vi "2100_Test_Guardian Switch_w Config.vi"(0 "Semiconductor Module Context":T7, 1 "SMU Current Settings":T6={"OFF_Current  Range"=1e-05, "OFF_Current  Level"=-1e-05, "ON_Current  Range"=0.001, "ON_Current  Level"=0.001} {"ON_Current  Level" format="%#_6p"; "ON_Current  Range" format="%#_6p"; "OFF_Current  Level" format="%#_6p"; "OFF_Current  Range" format="%#_6p"}, 2 "Master_Register_Data_Array_In":T1 {"Address" format="%.0x"}, 3 "Set_Meas_Sense":i32(ring)=1008 items=["Local"=1008, "Remote"=1009], 5 "Script_Info":T4={"Script Name"="WalkingState", "All_Scripts"=[]}, 7 "Publishable IDs":string[](array[string])=["LowPower", "Active"], 9 "USID":T3 max=15, 11 "Error In":errorcluster, 12 "Instrument_Pins":T5={"SMU_Pins"=["RF1", "RF2", "RF3", "RF4"], "HSDIO_Pins"=["CLK", "SDA"]}, 13 "Reg_Map_Bit_Name":string="RFC_SH", 14 "Reg_Map":string[][](array[string])=[["Reg Addr(0x00)", "7", "6", "5", "4", "3", "2", "1", "0"], ["0", "SPARE", "RF3_SH", "RF2_SH", "RF1_SH", "SPARE", "RF3_RFC", "RF2_RFC", "RF1_RFC"], ["1", "SPARE[7:0]", "", "", "", "", "", "", ""], ["2", "VVAR_EN", "LCM_EN", "RFC_SH", "SPARE", "VARACTOR[3:0]", "", "", ""], ["3", "SW_CTRL1_VIRTUAL[7:0]", "", "", "", "", "", "", ""], ["4", "SW_CTRL1_SWAP", "SW_CTRL1_RBSHIFT[2:0]", "", "", "SW_CTRL1_VSID[3:0]", "", "", ""], ["5", "REG_00_VIRTUAL_MASK[7:0]", "", "", "", "", "", "", ""], ["6", "LOCK_STATUS[1:0]", "", "CLK_DITHER", "FUSES_BURNED", "CLK_IDAC_CAL[3:0]", "", "", ""], ["7", "SPARE[2:0]", "", "", "ODFT_TRIM[4:0]", "", "", "", ""], ["8", "SPARE[2:0]", "", "", "HV_TRIM[4:0]", "", "", "", ""], ["9", "TEST_MUX[2:0]", "", "", "SPARE[1:0]", "", "MEMS_BG_TC[1:0]", "", "MEMSCP_RCM"], ["A", "CP_BOOST_OVRD_EN", "SPARE[2:0]", "", "", "PS_OFF_TIMER[1:0]", "", "PS_ON_TIMER[1:0]", ""], ["0", "", "", "", "", "", "", "", ""], ["D", "Reserved[1:0]", "", "WD_HI_EVENT_CNT[5:0]", "", "", "", "", ""], ["E", "VERSION_ID[7:0]", "", "", "", "", "", "", ""], ["F", "Reserved", "COUNT_200_LSB[6:0]", "", "", "", "", "", ""], ["10", "CLK_DIV2_EN", "Spare", "ODFT_EN", "HV_HYST[4:0]", "", "", "", ""], ["0", "", "", "", "", "", "", "", ""], ["12", "SHORT_FUSE", "FUSE_BURN", "STROBE_EN", "VIO_OK", "RTH[1:0]", "", "FUSE_LOAD_MAN_EN", "FUSE_LOAD"], ["13", "RR_ACK_EN", "Reserved", "ACK_POSITION[1:0]", "", "SuBUS_DRIVE_STRENGTH[3:0]", "", "", ""], ["14", "TM_IO_EN", "TM_IO_SEL", "SuBUS_OVS[1:0]", "", "Reserved[3:0]", "", "", ""], ["15", "Reserved[4:0]", "", "", "", "", "SuBUS_VERSION_PRESENT", "SuBUS_VOLTAGE", "SuBUS_FLAVOR_DEF"], ["16", "PROG_STROBE1_DUR[7:0]", "", "", "", "", "", "", ""], ["17", "PROG_STROBE0_DUR[7:0]", "", "", "", "", "", "", ""], ["18", "Reserved[2:0]", "", "", "EFUSE_SINGLE_ADDR_SEL[4:0]", "", "", "", ""], ["19", "POLL_ADR[4:0]", "", "", "", "", "POLL_BC[2:0]", "", ""], ["1A", "SOFTWARE_RESET", "Reserved[6:0]", "", "", "", "", "", ""], ["1B", "Reserved[7:0]", "", "", "", "", "", "", ""], ["1C", "PWR_MODE_1", "PWR_MODE_0", "TRIGGER_MASK[2:0]", "", "", "TRIGGER[2:0]", "", ""], ["1D", "PRODUCT_ID[7:0]", "", "", "", "", "", "", ""], ["1E", "MANUFACTURER_ID_LSB[7:0]", "", "", "", "", "", "", ""], ["1F", "MANUFACTURER_ID_MSB[3:0]", "", "", "", "USID[3:0]", "", "", ""]]) -> (6 "Master_Register_Data_Array_Out":T1 {"Address" format="%.0x"}, 15 "Error Out":errorcluster)   [LabVIEW 2013]
uses:
  Controls/USID.ctl
  <vilib>/NI_TestStand_SemiconductorModule/NI_TestStand_Semiconductor_Module.lvlibp/PinMap/General/SemiconductorModuleContext.ctl
  Controls/Master_Reg_Data_Array.ctl
  Controls/Reg_Address_Data.ctl
  <vilib>/NI_TestStand_SemiconductorModule/NI_TestStand_Semiconductor_Module.lvlibp/PinMap/DC Power/PinsToNIDCPowerSessions.vi
  <vilib>/NI_TestStand_SemiconductorModule/NI_TestStand_Semiconductor_Module.lvlibp/PinMap/General/Publish/PublishDataDoubleFunctionalTest.vi
  <vilib>/NI_TestStand_SemiconductorModule/NI_TestStand_Semiconductor_Module.lvlibp
panel:
  out "R Array":dbl[][](array[numeric]) format="%#_6p"
  in  "Tab Control":enum32{"Test Info", "Instrument Settings"}(tab)
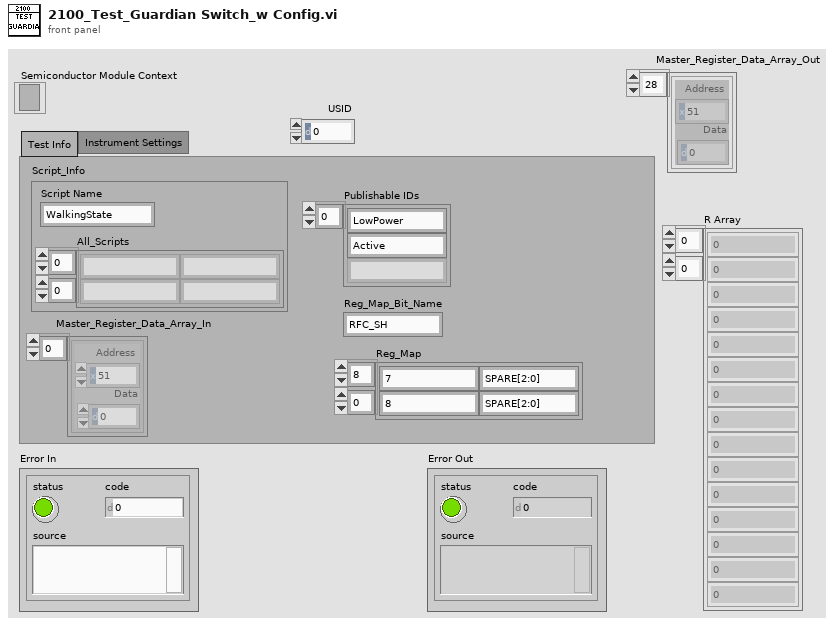
[diagram p1: front panel]
types:
  T1 = typedef "Master_Reg_Data_Array.ctl" = T2[]
  T2 = typedef "Reg_Address_Data.ctl" = cluster{"Address":u8, "Data":u8}
  T3 = typedef "USID.ctl" = u8
  T4 = cluster{"Script Name":string, "All_Scripts":string[][]}
  T5 = cluster{"SMU_Pins":string[], "HSDIO_Pins":string[]}
  T6 = cluster{"OFF_Current  Range":dbl, "OFF_Current  Level":dbl, "ON_Current  Range":dbl, "ON_Current  Level":dbl}
  T7 = typedef "NI_TestStand_Semiconductor_Module.lvlibp/SemiconductorModuleContext.ctl" = refnum<k7>
  T8 = typedef "Script Functions_Array.ctl" = enum16{"Reg_Write", "Bit_Write", "Delay", "Read", "Measure"}[]
  T9 = enum16{"Reg_Write", "Bit_Write", "Delay", "Read", "Measure"}
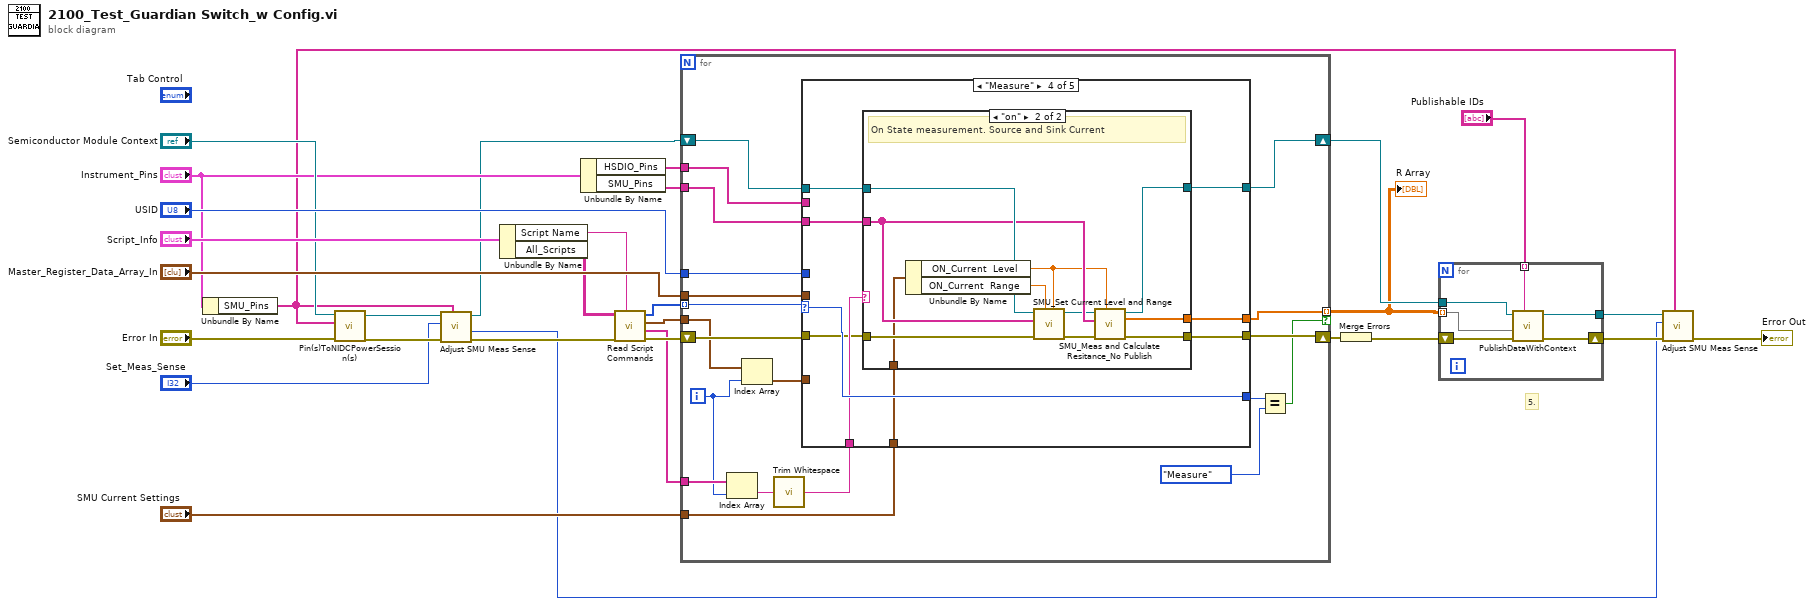
[diagram p0: block diagram]
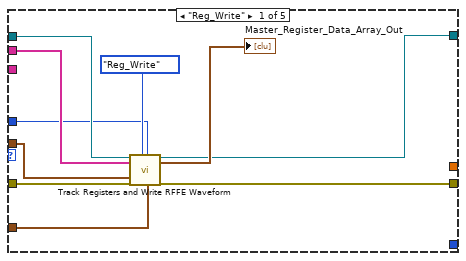
[diagram p2: hidden frame]
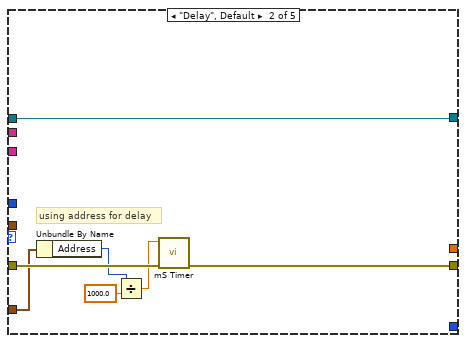
[diagram p3: hidden frame]
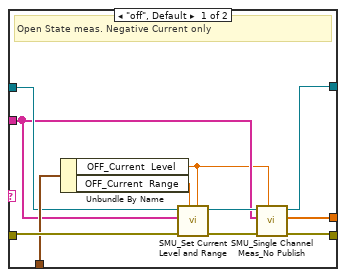
[diagram p5: hidden frame]
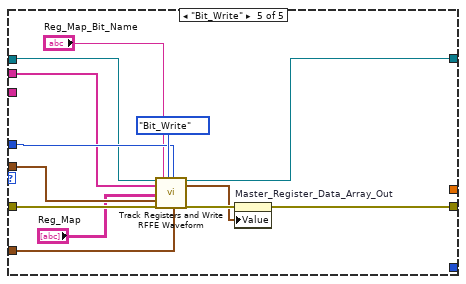
[diagram p6: hidden frame]
diagram:
  # "5."
  n1 = Unbundle By Name("Instrument_Pins") -> ("SMU_Pins"=w1:string[])
  n2 = call-poly <vilib>:"Pin(s)ToNIDCPowerSession(s).vi"("error in (no error)"="Error In", "Pins"=w1, "Semiconductor Module Context"="Semiconductor Module Context") -> ("error out"=w10:errorcluster, "Semiconductor Module Context Out"=w8:T7)  [unwired: 4 in, 3 out]
  n3 = call "Adjust SMU Meas Sense.vi"("Pins"=w1, "error in (no error)"=w10, "Set_Meas_Sense"="Set_Meas_Sense", "Semiconductor Module Context"=w8) -> ("error out"=w9:errorcluster, "Measurement:Sense"=w3:i32, "Semiconductor Module Context Out"=w7:T7)  [unwired: 5 in]
  n4 = Unbundle By Name("Script_Info") -> ("Script Name"=w20:string, "All_Scripts"=w21:string[][])
  n5 = Unbundle By Name("Instrument_Pins") -> ("HSDIO_Pins"=w24:string[], "SMU_Pins"=w23:string[])
  n6 = call "Read Script Commands.vi"("Test Name"=w20, "Error In"=w9, "All_Scripts"=w21) -> ("Error Out"=w27:errorcluster, "Script_Note"=w16:string[], "Script_Data"=w28:T2[], "Script_Functions"=w29:T8)  [unwired: 5 in]
  n7 = for {
    tunnel: "USID" -> [w45]
    tunnel: w29 -> [w44] mode=indexing
    tunnel: w28 -> [w48]
    tunnel: w24 -> [w49]
    shift-right: [w43] -> w25
    shift-left: w27 -> [w50]
    tunnel: "Master_Register_Data_Array_In" -> [w46]
    tunnel: w23 -> [w42]
    tunnel: [w31] -> w14 mode=indexing if=w38
    shift-right: [w41] -> w18
    shift-left: w7 -> [w37]
    tunnel: w16 -> [w36]
    tunnel: "SMU Current Settings" -> [w32]
    i -> [w35]
    n8 = Index Array(array=w36, index=w35) -> (element=w34:string)
    n9 = Index Array(array=w48, index=w35) -> (element=w47:T2)
    n10 = call <vilib>:"Trim Whitespace.vi"("string"=w34) -> ("trimmed string"=w33:string)  [unwired: 1 in]
    n11 = case shown="\"Measure\"" w44 {
      selector: w44 -> [_ _ _ w78 _]
      tunnel: w47 -> [w55 w66 _ _ w106]
      tunnel: w50 -> [w60 w67 w69 w76 w113]
      tunnel: w45 -> [w52 _ _ _ w111]
      tunnel: w37 -> [w58 w61 w68 w74 w110]
      tunnel: w49 -> [w57 _ _ _ w109]
      tunnel: [w59 w65 w69 w70 w103] -> w43
      tunnel: w46 -> [w54 _ _ _ w107]
      tunnel: w42 -> [_ _ _ w72 _]
      tunnel: [w51 w61 w68 w73 w101] -> w41
      tunnel: [_ _ _ w78 _] -> w40
      tunnel: w33 -> [_ _ _ w77 _]
      tunnel: w32 -> [_ _ _ w75 _]
      tunnel: [_ _ _ w71 _] -> w31
      frame "Reg_Write" {
        n12 = call "Track Registers and Write RFFE Waveform.vi"("Semiconductor Module Context"=w58, "Pins"=w57, "Master_Register_Data_Array_In"=w54, "Error In"=w60, "Script_Functions"=enum16{"Reg_Write", "Bit_Write"}."Reg_Write", "USID"=w52, "Reg_Address_Data"=w55) -> ("Semiconductor Module Context Out"=w51:T7, "Master_Register_Data_Array_Out"=→"Master_Register_Data_Array_Out":T1, "Error Out"=w59:errorcluster)  [unwired: 10 in]
      }
      frame "Delay", Default {
        # "using address for delay"
        n13 = Unbundle By Name(w66) -> ("Address"=w63:u8)
        n14 = Divide(x=w63, y=1000.0) -> (x/y=w62:dbl)
        n15 = call "mS Timer.vi"("Error In"=w67, "Delay(S)"=w62) -> ("Error Out"=w65:errorcluster)  [unwired: 9 in]
      }
      frame "Read" {
      }
      frame "Measure" {
        n16 = case shown="\"on\"" w77 {
          tunnel: w76 -> [w86 w99]
          tunnel: w75 -> [w85 w92]
          tunnel: w74 -> [w84 w95]
          tunnel: [w83 w97] -> w73
          tunnel: w72 -> [w82 w94]
          tunnel: [w80 w96] -> w71
          tunnel: [w79 w98] -> w70
          frame "off", Default {
            # "Open State meas. Negative Current only"
            n17 = Unbundle By Name(w85) -> ("OFF_Current  Level"=w81:dbl, "OFF_Current  Range"=w89:dbl)
            n18 = call "SMU_Set Current Level and Range.vi"("current level"=w81, "current range"=w89, "error in (no error)"=w86, "Pins"=w82, "Semiconductor Module Context"=w84) -> ("error out"=w88:errorcluster, "Semiconductor Module Context Out"=w87:T7)  [unwired: 5 in]
            n19 = call "SMU_Single Channel Meas_No Publish.vi"("Meas_A_Level"=w81, "error in (no error)"=w88, "Pins"=w82, "Semiconductor Module Context"=w87) -> ("error Out"=w79:errorcluster, "R Array"=w80:dbl[], "Semiconductor Module Context Out"=w83:T7)  [unwired: 5 in]
          }
          frame "on" {
            # "On State measurement. Source and Sink Current"
            n20 = Unbundle By Name(w92) -> ("ON_Current  Level"=w90:dbl, "ON_Current  Range"=w91:dbl)
            n21 = call "SMU_Set Current Level and Range.vi"("current level"=w90, "current range"=w91, "error in (no error)"=w99, "Pins"=w94, "Semiconductor Module Context"=w95) -> ("error out"=w100:errorcluster, "Semiconductor Module Context Out"=w93:T7)  [unwired: 5 in]
            n22 = call "SMU_Meas and Calculate Resitance_No Publish.vi"("Current  Level"=w90, "error in (no error)"=w100, "Pins"=w94, "Semiconductor Module Context"=w93) -> ("error Out"=w98:errorcluster, "R Array"=w96:dbl[], "Semiconductor Module Context Out"=w97:T7)  [unwired: 5 in]
          }
        }
      }
      frame "Bit_Write" {
        n23 = call "Track Registers and Write RFFE Waveform.vi"("Semiconductor Module Context"=w110, "Pins"=w109, "Reg_Map"="Reg_Map", "Master_Register_Data_Array_In"=w107, "Error In"=w113, "Reg_Map_Bit_Name"="Reg_Map_Bit_Name", "Script_Functions"=enum16{"Reg_Write", "Bit_Write"}."Bit_Write", "USID"=w111, "Reg_Address_Data"=w106) -> ("Semiconductor Module Context Out"=w101:T7, "Master_Register_Data_Array_Out"=w102:T1, "Error Out"=w104:errorcluster)  [unwired: 8 in]
        n24 = property on="Master_Register_Data_Array_Out" class="Arr (strict)"(error in=w104, "Value"=w102) -> (error out=w103:errorcluster)  [unwired: 1 in, 1 out]
      }
    }
    n25 = Equal?(x=w40, y=T9."Measure" ("Enum")) -> (x = y?=w38:bool)
  }
  "R Array" <- w14
  n26 = Merge Errors(w25) -> (w19:errorcluster)
  n27 = for {
    shift-right: [w119] -> w5
    shift-left: w19 -> [w118]
    tunnel: w18 -> [w117]
    tunnel: "Publishable IDs" -> [w116] mode=indexing
    tunnel: w14 -> [w115] mode=indexing
    tunnel: [w114] -> w2
    n28 = call-poly <vilib>:"PublishDataWithContext.vi"("Published Data Id"=w116, "error in (no error)"=w118, "Data In"=w115, "Semiconductor Module Context"=w117) -> ("error out"=w119:errorcluster, "Semiconductor Module Context Out"=w114:T7)  [unwired: 6 in]
  }
  n29 = call "Adjust SMU Meas Sense.vi"("Pins"=w1, "error in (no error)"=w5, "Set_Meas_Sense"=w3, "Semiconductor Module Context"=w2) -> ("error out"=→"Error Out":errorcluster)  [unwired: 5 in, 2 out]
